vi "TCP-Set AO Gains.vi"(8 "error in (no error)":errorcluster, 10 "Gain String":string, 11 "Channel String":string) -> (0 "error out":errorcluster)   [LabVIEW 2015]
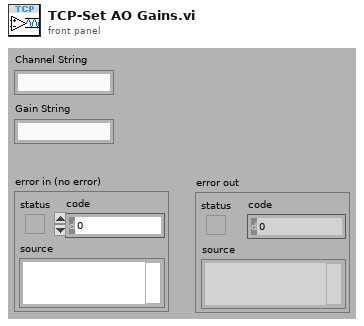
[diagram p1: front panel]
types:
  T1 = enum16{"Init", "Write", "Read", "Latch setup", "Compute comp."}
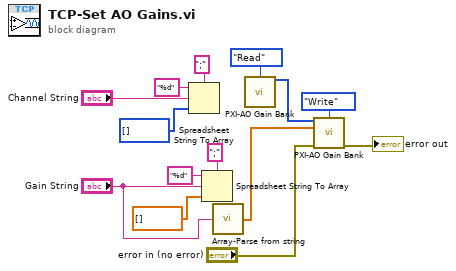
[diagram p0: block diagram]
diagram:
  n1 = Spreadsheet String To Array(delimiter (Tab)=";", format string="%d", spreadsheet string="Channel String", array type (2D Dbl)=i32[] []) -> ()  [unwired: 1 out]
  n2 = Spreadsheet String To Array(delimiter (Tab)=";", format string="%d", spreadsheet string="Gain String", array type (2D Dbl)=dbl[] []) -> ()  [unwired: 1 out]
  n3 = call "Array-Parse from string.vi"("String"="Gain String") -> ("Array"=w1:dbl[])  [unwired: 13 in, 1 out]
  n4 = call "PXI-AO Gain Bank.vi"("Action"=T1."Read") -> ("Channels"=w3:i32[])  [unwired: 9 in, 5 out]
  n5 = call "PXI-AO Gain Bank.vi"("AO Channels"=w3, "Action"=T1."Write", "Gains"=w1, "error in (no error)"="error in (no error)") -> ("error out"=→"error out":errorcluster)  [unwired: 6 in, 5 out]
